vi "Dashboard Main.vi"() -> ()   [LabVIEW 2016]
uses:
  <vilib>/Utility/miscctls.llb/LVRowAndColumnTypeDef.ctl
  <vilib>/event_ctls.llb/eventvkey.ctl
  <vilib>/Utility/file.llb/Read Delimited Spreadsheet (DBL).vi
  <vilib>/Utility/file.llb/Write Delimited Spreadsheet (DBL).vi
  <vilib>/Rock Robotics/Network Tables/NT Write Boolean.vi
  <vilib>/Rock Robotics/Network Tables/NT Read Numeric Array.vi
  <vilib>/Rock Robotics/WPI/Dashboard/WPI_DashboardLogging Global.vi
panel:
  out "error out":errorcluster
  out "error out 2":errorcluster
  in  "Camera Settings Right":T1={"Frame Rate"=30, "Compression"=30, "Size"=1, "DB Camera Config"=FALSE} {"Frame Rate" scale=1.0..30.0; "Compression" scale=100.0..-1.0; "Size" items=["640x480", "320x240", "160x120"]}
  in  "Camera Name Right":string(combo)="No Camera Selection"
  out "Camera Info":cluster{"Mbps LED":bool, "Mbps":dbl, "fps":dbl} {"fps" format="%#.1g"; "Mbps" format="%#.1g"}
  in  "Camera Settings":T1={"Frame Rate"=30, "Compression"=30, "Size"=1, "DB Camera Config"=FALSE} {"Frame Rate" scale=1.0..30.0; "Compression" scale=100.0..-1.0; "Size" items=["640x480", "320x240", "160x120"]}
  in  "TCP":refnum<k5>
  in  "Rec Mode":enum32{"Stop", "Record", "Playback"}(radio)
  out "Robot IP":string
  out "Image Message":string="Timeout in Camera Communications"
  in  "Dashboard Tab":T2(tab)
  in  "Mode":bool
  in  "Select Auto":string(combo)="Select Autonomous ..."
  out "NT Connection":bool
  out "MotorChart R":cluster{"Numeric":dbl, "Numeric":dbl}(graph)
  out "MotorChart L":cluster{"Numeric":dbl, "Numeric":dbl}(graph)
  out "MotorSliders R":cluster{"MotorSlide1":dbl, "MotorSlide2":dbl} {"MotorSlide2" scale=-1.0..1.0 scale format="%#_2e"; "MotorSlide1" scale=-1.0..1.0 scale format="%#_2e"}
  out "MotorSliders L":cluster{"MotorSlide1":dbl, "MotorSlide2":dbl} {"MotorSlide2" scale=-1.0..1.0 scale format="%#_2e"; "MotorSlide1" scale=-1.0..1.0 scale format="%#_2e"}
  out "JS1 Z":dbl(slide) scale=-1.0..1.0 scale format="%#_2e"
  out "JS1 Graph":cluster{"X":dbl, "Y":dbl}[](graph)
  out "JS1 Buttons":T3
  out "JS2 Z":dbl(slide) scale=-1.0..1.0 scale format="%#_2e"
  out "JS2 Graph":cluster{"X":dbl, "Y":dbl}[](graph)
  out "JS2 Buttons":T3
  out "Mode":T4(ring)=enum."Auto Disabled"
  out "Gear State":string="Waiting...."
  out "Camera Image Right":T5(plugin-control)
  in  "Test Slider":dbl(slide) scale=0.0..100.0 scale format="%#_3g"
  in  "On/Off":bool caption="Solenoid"
  in  "Test Name":u16(ring) items=["Select the test to run..."]
  in  "Test Tree":string(tree)
  in  "Motor":cluster{"Value":dbl, "Enable":bool} {"Value" scale=-1.0..1.0 scale format="%#_3g"}
  out "Progress":T6 {"Test Progress" scale=0.0..100.0}
  in  "Rev/Fwd":cluster{"Forward":bool, "Reverse":bool}
  in  "Test Ring":u16(ring) items=["Monochrome", "Color"]
  out "Cmd Status":string
  in  "Execute Command":bool
  in  "Command Params":string[][](table)
  in  "Command Selection":i32(listbox)
  in  "CheckList":i32(listbox)
  out "Tree":string(tree)
  in  "Max Speed":dbl=1.0 format="%#_13g"
  in  "Foreward Sensitivity":dbl=1.0 format="%#_13g"
  in  "Turning Sensitity":dbl=0.4 format="%#_13g"
  in  "High Gear Turning Multiplier":dbl=0.65 format="%#_13g"
  in  "Save":bool
  in  "Load":bool
  in  "Autoshift":bool=TRUE
  in  "Direction Toggle":bool=TRUE
  in  "High Gear":bool=TRUE
  in  "Profile Name":string="Profile1"
  out "Camera Image":T5(plugin-control)
  out "Background":bool
  in  "Camera Name":string(combo)="No Camera Selection"
  # "HW"
  # "HW"
  # "Joysticks"
  # "This is the number that is multiplied with the joystick output to determine high gear turning speed, the lower the number the slower it will turn in high gear."
  # "These numbers controls overall how sensitive the joystick is to turning and foreward movement, the lower the number is the faster it will respond to joystick motion. \nIf the number is 1 then it will move in a linear relationship with the joystick."
  # "This controls the maximum foreward and backwards speed of the robot, if at 1 then the robot can move at max power, if at 0 then the robot cannot move at all."
  # "This turns the ability to use autoshift on/off, if activated it does NOT mean that autoshift is always on, it simply means that it can be turned on with buttons 6/11."
  # "This turns the ability to use high gear on/off, if activated it does NOT mean that high gear is always on, it simply means that it can be turned on with button 1."
  # "This turns on the ability to reverse the direction of the robot with the buttons 8/9."
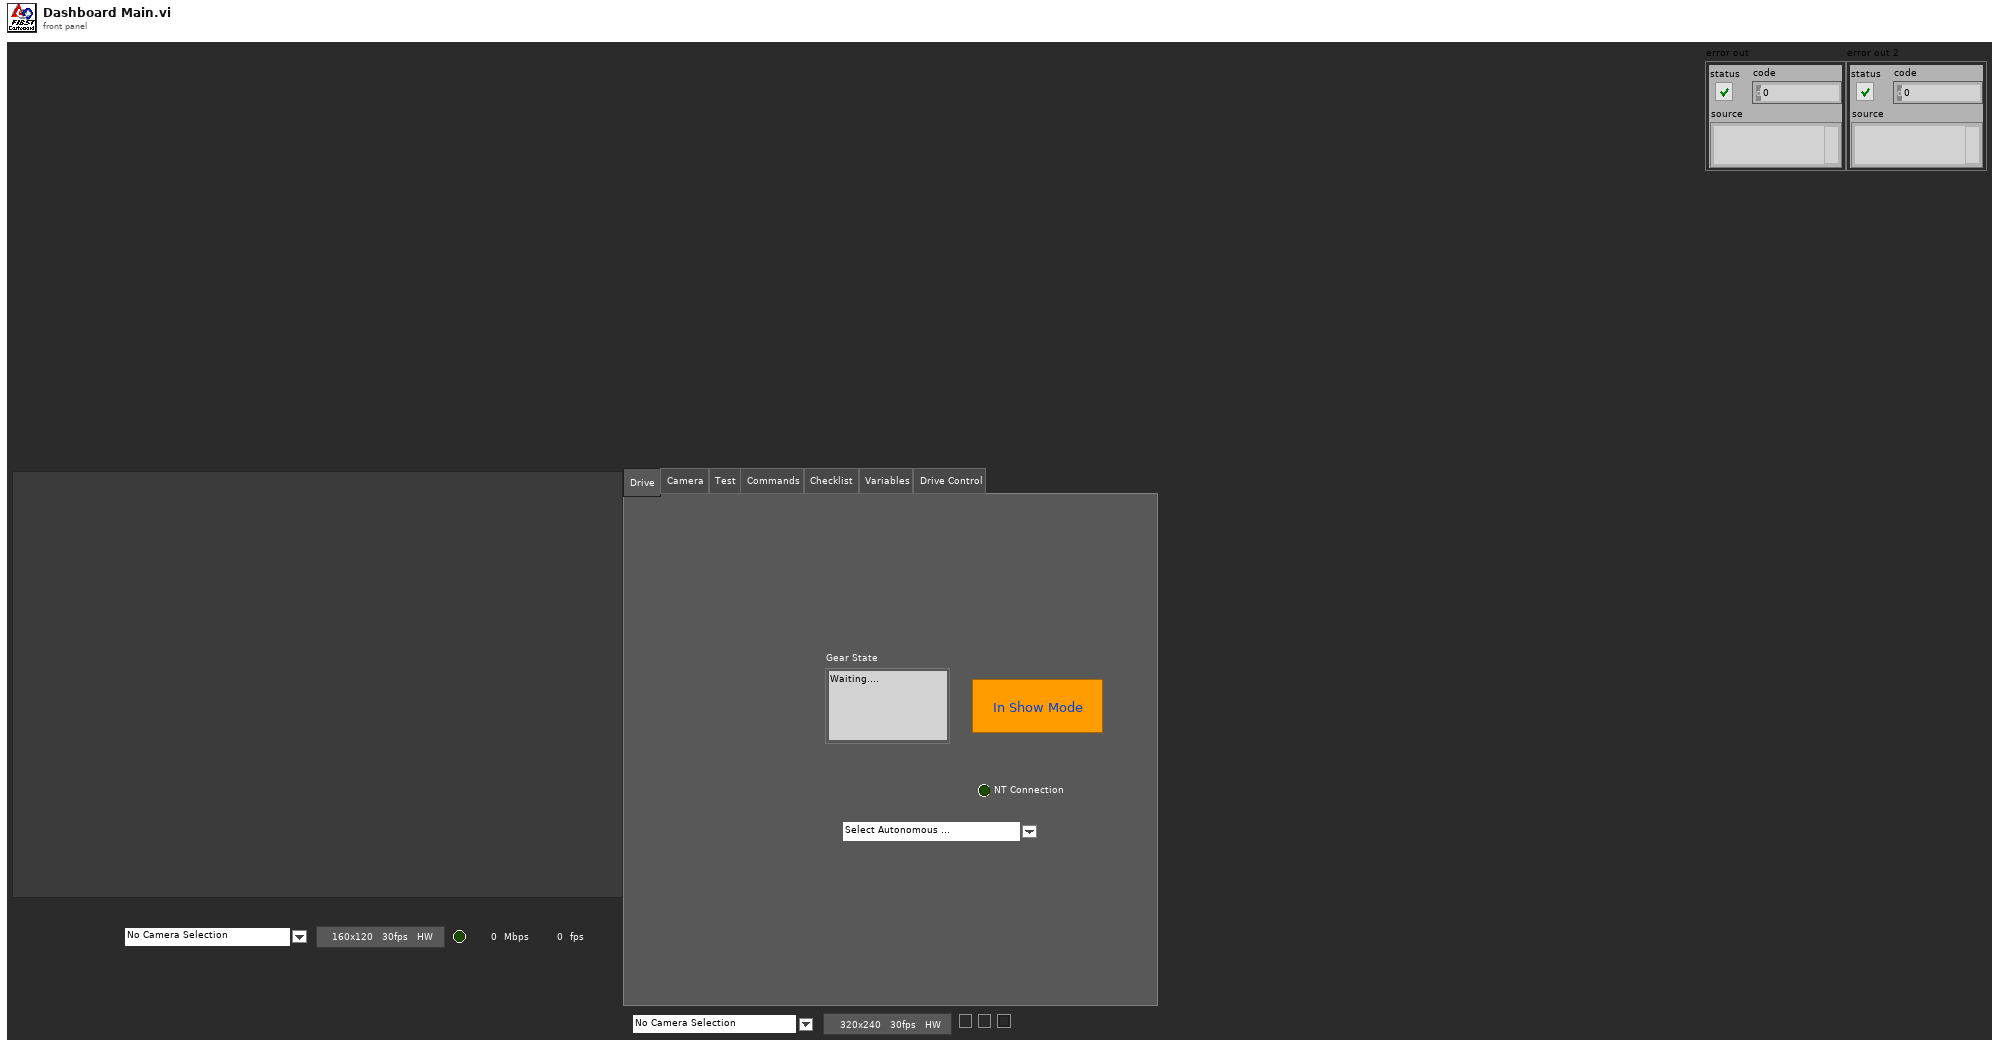
[diagram p1: front panel]
types:
  T1 = cluster{"Frame Rate":i32, "Compression":i32, "Size":u16, "DB Camera Config":bool}
  T2 = enum32{"Drive", "Camera", "Basic", "Custom", "Test", "Commands", "Checklist", "Variables", "Drive Control"}
  T3 = cluster{bool, bool, bool, bool, bool, bool, bool, bool, bool, bool, bool, bool}
  T4 = enum8{"Tele-Op Disabled", "Tele-Op Enabled", "Auto Disabled", "Auto Enabled", "Test Disabled", "Test Enabled", "Disconnected", "No Code", "E-Stop"}
  T5 = typedef "IMAQ Image.ctl" = refnum<image>
  T6 = cluster{"Test Progress":u8, "Test Progress Text":string}
  T7 = typedef "Image Type" = u32
  T8 = cluster{"IDs":cluster{"RPC field ID":u16, "Unique ID":u16}, "String":string}
  T9 = enum32{"Drive", "Camera", "Basic", "Custom", "Test", "Commands", "Checklist", "Variables"}
  T10 = enum32{"Drive", "Basic", "Custom", "Test", "Checklist", "Variables"}
  T11 = cluster{"Error Strings":string, "Disable Counts":cluster{u16, u16}, "Rail Faults":cluster{u16, u16, u16}, "Robot IP":string, "DB Mode":u8, "Event Info":cluster{"Name":string, "Type":u8, "Number":u16, "Replay":u8}}
  T12 = cluster{"Storage":cluster{"Disk Free":u64, "RAM Block":u32, "RAM free":u32}, "CPU Utilization":cluster{"CPU % ISR":sgl, "CPU % Time Crit":sgl, "CPU % Timed Str":sgl, "CPU % High":sgl, "CPU % Above":sgl, "CPU % Normal":sgl, "CPU % Low":sgl}, "CAN":cluster{"% Bus Utilization":sgl, "Bus Off Cnt":u32, "TX_FIFO Full Cnt":u32, "Receive Error Cnt":u8, "Transmit Error Cnt":u8}, "HID":cluster{"HID Outputs":u32, "Rumble Low":u16, "Rumble High":u16}[]}
  T13 = cluster{"Status bits":cluster{"Test Mode":bool, "Autonomous":bool, "Enabled":bool, "Code Start":bool, "Brownout":bool, "Reserved 2":bool, "Reserved 3":bool, "E-Stop":bool}, "Code Trace":cluster{"Disabled":bool, "TeleOp":bool, "Auto":bool, "Test":bool}, "Controller Type":enum16{"unknown", "cRIO", "roboRio"}, "Code?":enum16{"unknown", "noCode", "code"}, "Battery V":dbl}
  T14 = cluster{"Control Bits":cluster{"TestMode":bool, "Autonomous":bool, "Enabled":bool, "FMS Present":bool, bool, bool, bool, "E-Stop":bool}, "Team Station ":u8, "Countdown":sgl, "Joystick Values":cluster{"Axes":dbl[], "Buttons":bool[], "POVs":i16[]}[]}
  T15 = cluster{"Axes":dbl[], "Buttons":bool[], "POVs":i16[]}[]
  T16 = cluster{"Axes":dbl[], "Buttons":bool[], "POVs":i16[]}
  T17 = cluster{"Buttons[0]":bool, "Buttons[1]":bool, "Buttons[2]":bool, "Buttons[3]":bool, "Buttons[4]":bool, "Buttons[5]":bool, "Buttons[6]":bool, "Buttons[7]":bool, "Buttons[8]":bool, "Buttons[9]":bool, "Buttons[10]":bool, "Buttons[11]":bool}
  T18 = cluster{"Camera Image":refnum<vi>, "Dashboard Tab":refnum<vi>, "Background":refnum<vi>, "Rec Mode":refnum<vi>, "Test Slider":refnum<vi>, "On/Off ":refnum<vi>, "Test Ring":refnum<vi>, "Rev/Fwd":refnum<vi>, "Test Name":refnum<vi>, "Motor":refnum<vi>, "Progress":refnum<vi>, "CheckList":refnum<vi>, "Tree":refnum<vi>, "Test Tree":refnum<vi>, "Command Params":refnum<vi>, "Command Selection":refnum<vi>, "Execute Command":refnum<vi>, "Cmd Status":refnum<vi>, "Camera Settings":refnum<vi>, "Camera Name":refnum<vi>, "Camera Info":refnum<vi>, "Camera Settings Right":refnum<vi>, "Camera Name Right":refnum<vi>, "Camera Image Right":refnum<vi>}
  T19 = cluster{"Operation":enum16{"Update", "Clear"}, "Color Box":u32}[]
  T20 = typedef "eventvkey.ctl" = enum16{"ASCII", "Enter", "Return", "Shift", "Ctrl", "Alt", "Cmd", "Opt", "Caps", "NumLock", "Clear", "Break", "Up", "Down", "Left", "Right", "Insert", "Delete", "Home", "End", "PageUp", "PageDown", "Escape", "Help", "Pause", "ScrollLock", "F1", "F2", "F3", "F4", "F5", "F6", "F7", "F8", "F9", "F10", "F11", "F12", "F13", "F14", "F15", "F16", "F17", "F18", "F19", "F20", "F21", "F22", "F23", "F24", "Play", "VolumeUp", "VolumeDown", "Mute", "Two Byte Char"}
  T21 = cluster{"Image Size":bool, "Image Type":bool, "Pixel Value":bool, "ROI Information":bool, "Zoom Factor":bool}
  T22 = cluster{"Operation":enum16{"Update", "Clear"}, "Color Box":u32}
  T23 = typedef "LVRowAndColumnTypeDef.ctl" = cluster{"Row":i32, "Column":i32}
  T24 = cluster{"Shift":bool, "Ctrl":bool, "Alt":bool, "Cmd":bool, "Opt":bool}
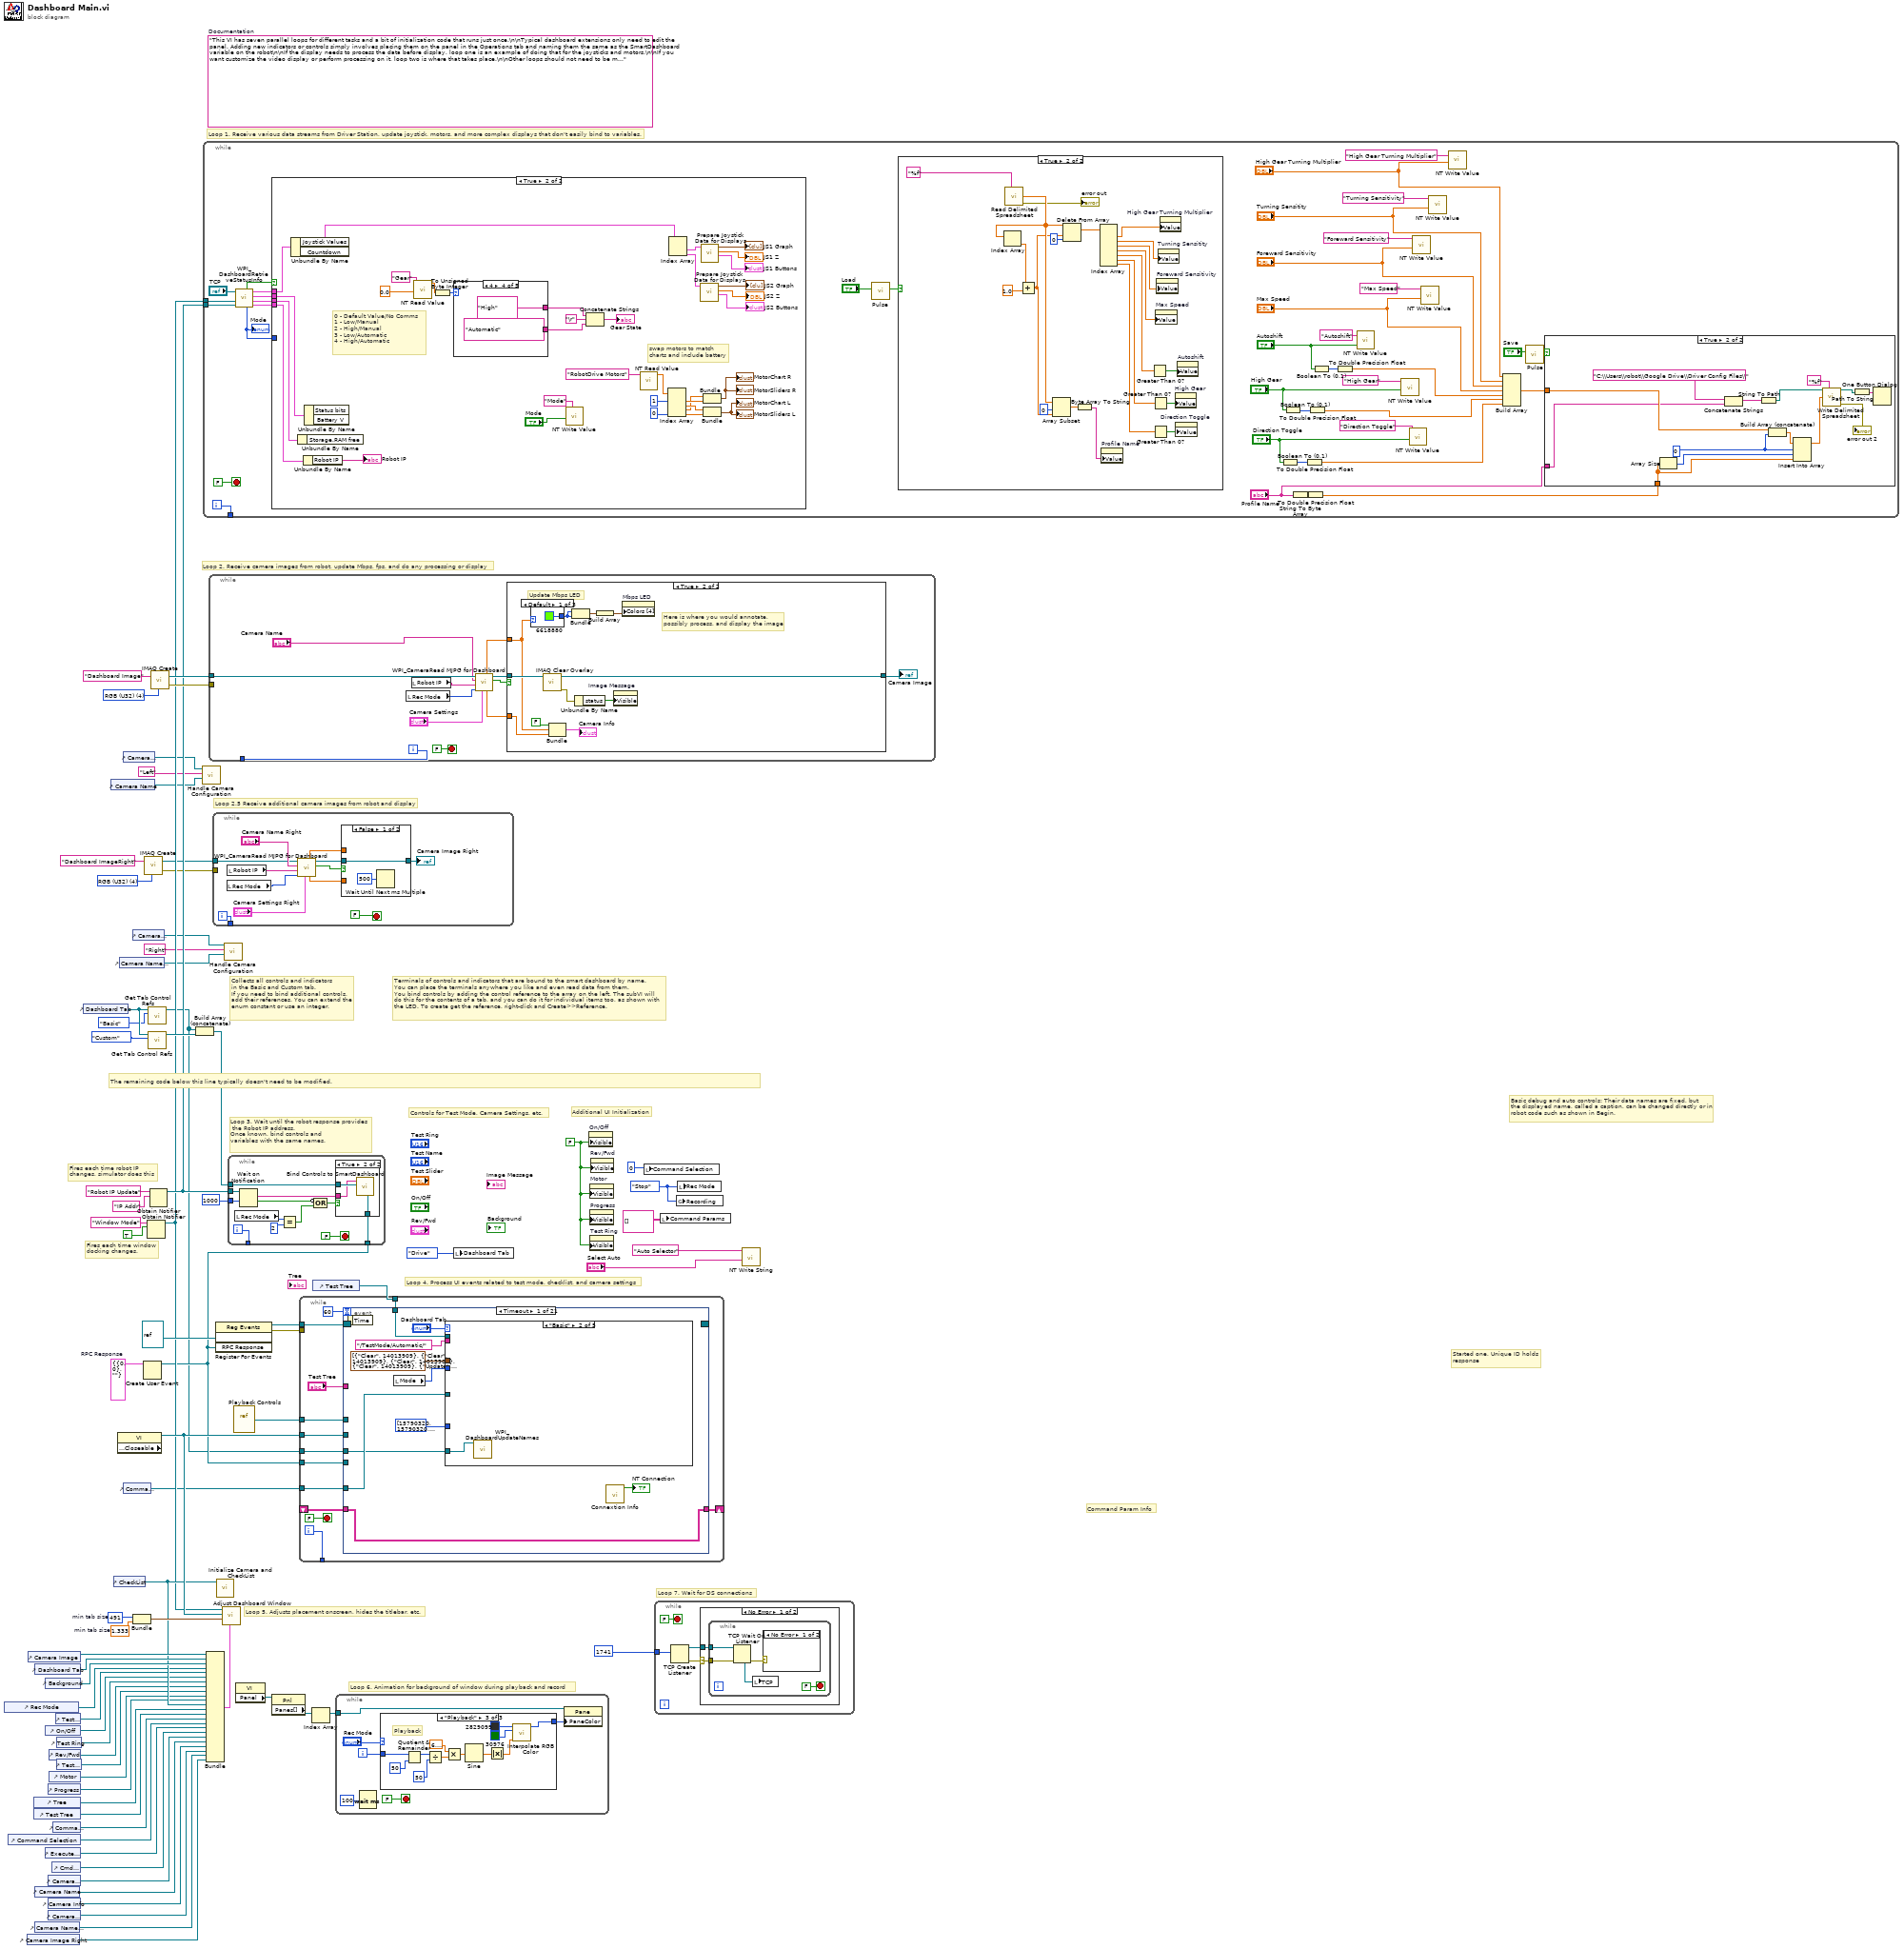
[diagram p0: block diagram]
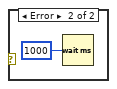
[diagram p3: hidden frame]
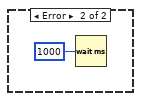
[diagram p4: hidden frame]
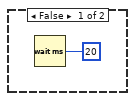
[diagram p7: hidden frame]
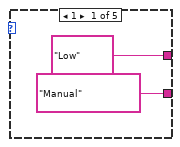
[diagram p8: hidden frame]
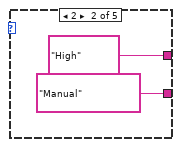
[diagram p9: hidden frame]
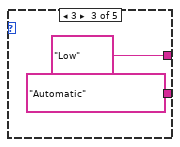
[diagram p10: hidden frame]
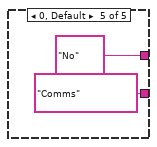
[diagram p11: hidden frame]
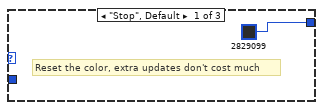
[diagram p12: hidden frame]
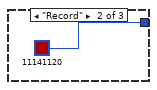
[diagram p13: hidden frame]
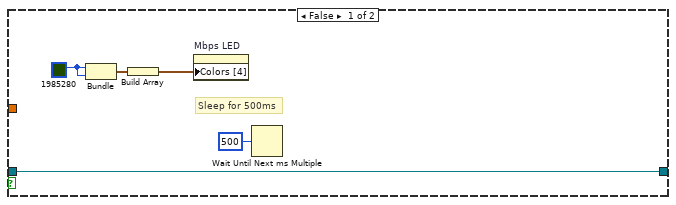
[diagram p15: hidden frame]
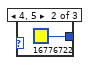
[diagram p16: hidden frame]
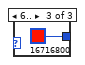
[diagram p17: hidden frame]
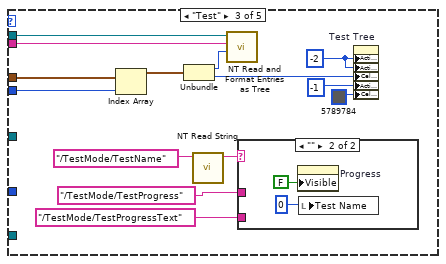
[diagram p19: hidden frame]
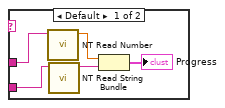
[diagram p20: hidden frame]
diagram:
  w10 = T7 4 items=["Grayscale (U8)", "Grayscale (I16)", "Grayscale (SGL)", "Complex (CSG)", "RGB (U32)", "HSL (U32)", "RGB (U64)"] ("Image Type")
  w26 = T8 {"IDs"={"RPC field ID"=0, "Unique ID"=0}, "String"=""}  # RPC Response
  w51 = 491  # min tab size
  w50 = 1.333  # min tab size
  w58 = enum32{"Stop", "Record", "Playback"}."Stop" ("Rec Mode")
  w33 = FALSE ("Visible")
  (unwired) "This VI has seven parallel loops for different tasks and a bit of initialization code that runs just once.\n\nTypical dashboard extensions only need to edit the panel. Adding new indicators or controls simply involves placing them on the panel in the Operations tab and naming them the same as the SmartDashboard variable on the robot\n\nIf the display needs to process the data before display, loop one is an example of doing that for the joysticks and motors.\n\nIf you want customize the video display or perform processing on it, loop two is where that takes place.\n\nOther loops should not need to be modified. They are pretty standard, and document the task they perform."  # Documentation
  w75 = T7 4 items=["Grayscale (U8)", "Grayscale (I16)", "Grayscale (SGL)", "Complex (CSG)", "RGB (U32)", "HSL (U32)", "RGB (U64)"] ("Image Type")
  # "Loop 2.5 Receive additional camera images from robot and display"
  # "Command Param Info"
  # "Started one, Unique ID holds\nresponse"
  # "Loop 7. Wait for DS connections"
  # "Basic debug and auto controls: Their data names are fixed, but\nthe displayed name, called a caption, can be changed directly or in\nrobot code such as shown in Begin."
  # "Controls for Test Mode, Camera Settings, etc."
  # "Additional UI Initialization"
  # "Loop 6. Animation for background of window during playback and record"
  # "Fires each time robot IP\nchanges, simulator does this"
  # "Fires each time window\ndocking changes."
  # "Collects all controls and indicators\nin the Basic and Custom tab.\nIf you need to bind additional controls,\nadd their references. You can extend the\nenum constant or use an integer."
  # "The remaining code below this line typically doesn't need to be modified."
  # "Loop 4. Process UI events related to test mode, checklist, and camera settings"
  # "Terminals of controls and indicators that are bound to the smart dashboard by name.\nYou can place the terminals anywhere you like and even read data from them.\nYou bind controls by adding the control reference to the array on the left. The subVI will\ndo this for the contents of a tab, and you can do it for individual items too, as shown with\nthe LED. To create get the reference, right-click and Create>>Reference."
  # "Loop 3. Wait until the robot response provides\n the Robot IP address.\nOnce known, bind controls and\nvariables with the same names."
  # "Loop 5. Adjusts placement onscreen, hides the titlebar, etc."
  # "Loop 1. Receive various data streams from Driver Station, update joystick, motors, and more complex displays that don't easily bind to variables."
  # "Loop 2. Receive camera images from robot, update Mbps, fps, and do any processing or display"
  n1 = control-ref of="Rec Mode"() -> (w39:refnum<vi>)
  n2 = control-ref of="Command Selection"() -> (w25:refnum<vi>)
  n3 = control-ref of="Camera Image Right"() -> (w1:refnum<vi>)
  n4 = control-ref of="Camera Image"() -> (w53:refnum<vi>)
  n5 = control-ref of="Tree"() -> (w43:refnum<vi>)
  n6 = control-ref of="Test Tree"() -> (w42:refnum<vi>)
  n7 = control-ref of="Dashboard Tab"() -> (w52:refnum<vi>)
  n8 = control-ref of="Camera Name"() -> (w16:refnum<vi>)
  n9 = control-ref of="Camera Name Right"() -> (w2:refnum<vi>)
  n10 = control-ref of="Execute Command"() -> (w27:refnum<vi>)
  n11 = control-ref of="Background"() -> (w48:refnum<vi>)
  n12 = control-ref of="On/Off"() -> (w37:refnum<vi>)
  n13 = control-ref of="Progress"() -> (w34:refnum<vi>)
  n14 = control-ref of="Camera Settings"() -> (w17:refnum<vi>)
  n15 = control-ref of="Camera Info"() -> (w15:refnum<vi>)
  n16 = control-ref of="Camera Settings Right"() -> (w3:refnum<vi>)
  n17 = control-ref of="Rev/Fwd"() -> (w35:refnum<vi>)
  n18 = control-ref of="Motor"() -> (w40:refnum<vi>)
  n19 = control-ref of="Cmd Status"() -> (w21:refnum<vi>)
  n20 = control-ref of="Command Params"() -> (w28:refnum<vi>)
  n21 = control-ref of="Test Slider"() -> (w38:refnum<vi>)
  n22 = control-ref of="Test Ring"() -> (w36:refnum<vi>)
  n23 = control-ref of="Test Name"() -> (w41:refnum<vi>)
  n24 = control-ref of="Dashboard Tab"() -> (w56:refnum<vi>)
  n25 = control-ref of="Camera Name"() -> (w18:refnum<vi>)
  n26 = control-ref of="CheckList"() -> (w44:refnum<vi>)
  n27 = property class="VI" props=["Front Panel.Closeable"]() -> (reference out=w57:refnum<vi>)  [unwired: 2 in, 2 out]
  n28 = control-ref of="Camera Name Right"() -> (w6:refnum<vi>)
  n29 = control-ref of="Camera Settings"() -> (w19:refnum<vi>)
  n30 = control-ref of="Command Params"() -> (w20:refnum<vi>)
  n31 = control-ref of="Camera Settings Right"() -> (w7:refnum<vi>)
  n32 = Bundle("min tab size"=w51, "min tab size"=w50) -> (w49:cluster{"min tab size":i32, "min tab size":dbl})  [unwired: 1 in]
  n33 = Create User Event(user event datatype=w26) -> (user event=w22:refnum<user-event>)  [unwired: 1 in, 1 out]
  n34 = call "IMAQ Create"("Image Name"="Dashboard ImageRight", "Image Type"=w10) -> ("New Image"=w9:T5, "error out"=w8:errorcluster)  [unwired: 2 in, 1 out]
  n35 = Obtain Notifier(name (unnamed)="Window Mode", notification data type=TRUE) -> (notifier out=w31:refnum<notifier>)  [unwired: 2 in, 2 out]
  n36 = call <vilib>:"Get Tab Control Refs.vi"("Page Index"=T10."Basic" ("Dashboard Tab"), "TabControl in"=w56) -> ("ControlsOnPage"=w14:refnum<vi>[])  [unwired: 9 in]
  n37 = call <vilib>:"Get Tab Control Refs.vi"("Page Index"=T10."Custom" ("Dashboard Tab"), "TabControl in"=w56) -> ("ControlsOnPage"=w55:refnum<vi>[])  [unwired: 9 in]
  n38 = Obtain Notifier(name (unnamed)="Robot IP Update", notification data type="IP Addr" ("name (unnamed)")) -> (notifier out=w32:refnum<notifier>)  [unwired: 2 in, 2 out]
  n39 = call "IMAQ Create"("Image Name"="Dashboard Image", "Image Type"=w75) -> ("New Image"=w73:T5, "error out"=w72:errorcluster)  [unwired: 2 in, 1 out]
  n40 = Build Array (concatenate)(w14, w55) -> (w54:refnum<vi>[])
  n41 = call "Handle Camera Configuration.vi"("CameraNameRef"=w18, "Camera File Name"="Left", "ClusterRef"=w19) -> ()  [unwired: 9 in]
  n42 = while {
    tunnel: [w113] -> _
    tunnel: w32 -> [w107]
    tunnel: w31 -> [w104]
    i -> [w113]
    stop <- FALSE stop-if-true
    n43 = call <vilib>:"WPI_DashboardRetrieveStatusInfo.vi"("Binding Refnum"=w107, "Window Mode Notifier"=w104, "TCP Cnx"="TCP") -> ("Power and Errors"=w108:T11, "Robot Metrics"=w111:T12, "Status Info"=w112:T13, "Control Info"=w109:T14, "Robot Mode"=w106:T4, "Process?"=w110:bool)  [unwired: 3 in]
    "Mode" <- w106
    n44 = case shown="True" w110 {
      tunnel: w112 -> [_ w184]
      tunnel: w111 -> [_ w183]
      tunnel: w109 -> [_ w182]
      tunnel: w108 -> [_ w181]
      tunnel: w106 -> [_ _]
      frame False {
        n45 = Wait (ms)(milliseconds to wait=u32 20) -> ()  [unwired: 1 out]
      }
      frame True {
        # "0 - Default Value/No Comms\n1 - Low/Manual\n2 - High/Manual\n3 - Low/Automatic\n4 - High/Automatic"
        # "swap motors to match\ncharts and include battery"
        n46 = Unbundle By Name(w182) -> ("Joystick Values"=w172:T15)  [unwired: 1 out]
        n47 = Unbundle By Name(w183) -> ()  [unwired: 1 out]
        n48 = Unbundle By Name(w181) -> ("Robot IP"=→"Robot IP":string)
        n49 = Unbundle By Name(w184) -> ()  [unwired: 2 out]
        n50 = call-poly <vilib>:"NT Read Value.vi"("Default Value"=0.0, "Name"="Gear") -> ("Numeric"=w160:dbl)  [unwired: 8 in, 1 out]
        n51 = To Unsigned Byte Integer(number=w160) -> (unsigned 8bit integer=w159:u8)
        n52 = case shown="4" w159 {
          tunnel: ["Low" "High" "Low" "High" "No"] -> w155
          tunnel: ["Manual" "Manual" "Automatic" "Automatic" "Comms"] -> w157
          frame 1 {
          }
          frame 2 {
          }
          frame 3 {
          }
          frame 4 {
          }
          frame 0, Default {
          }
        }
        n53 = call-poly <vilib>:"NT Write Value.vi"("Boolean"="Mode", "Name"="Mode") -> ()  [unwired: 9 in, 1 out]
        n54 = Concatenate Strings(w155, "\r", w157) -> (→"Gear State":string)
        n55 = call-poly <vilib>:"NT Read Value.vi"("Name"="RobotDrive Motors") -> ("Numeric Array"=w162:dbl[])  [unwired: 9 in, 1 out]
        n56 = Index Array(array=w162, index #1=1, index #4=0) -> (element #1=w176:dbl, element #2=w177:dbl, element #3=w175:dbl, element #4=w180:dbl)  [unwired: 2 in]
        n57 = Index Array(array=w172) -> (element #1=w171:T16, element #2=w167:T16)  [unwired: 2 in]
        n58 = call "Prepare Joystick Data for Displays.vi"("Joystick Values"=w167) -> ("Buttons"=→"JS2 Buttons":T17, "Z Axis"=→"JS2 Z":dbl, "Cartesian Data"=→"JS2 Graph":cluster{"X axis":dbl, "X axis":dbl}[])  [unwired: 8 in]
        n59 = call "Prepare Joystick Data for Displays.vi"("Joystick Values"=w171) -> ("Buttons"=→"JS1 Buttons":T17, "Z Axis"=→"JS1 Z":dbl, "Cartesian Data"=→"JS1 Graph":cluster{"X axis":dbl, "X axis":dbl}[])  [unwired: 8 in]
        n60 = Bundle("Numeric"=w175, "Numeric"=w176) -> (→"MotorChart R" →"MotorSliders R":cluster{"Numeric":dbl, "Numeric":dbl})  [unwired: 1 in]
        n61 = Bundle("Numeric"=w177, "Numeric"=w180) -> (→"MotorChart L" →"MotorSliders L":cluster{"Numeric":dbl, "Numeric":dbl})  [unwired: 1 in]
      }
    }
    n62 = call "Pulse.vi"("Input"="Load") -> ("Output"=w94:bool)  [unwired: 10 in]
    n63 = case shown="True" w94 {
      frame False {
      }
      frame True {
        n64 = call-poly <vilib>:"Read Delimited Spreadsheet.vi"("format (%.3f)"="%f") -> ("first row"=w132:dbl[], "error out"=→"error out":errorcluster)  [unwired: 9 in, 4 out]
        n65 = Index Array(array=w132) -> (element=w117:dbl)  [unwired: 1 in]
        n66 = Add(x=w117, y=1.0) -> (x+y=w116:dbl)
        n67 = Array Subset(array=w132, index=0, length=w116) -> (w133:dbl[])
        n68 = Delete From Array(array=w132, length=w116, index=0) -> (array with subset deleted=w130:dbl[])  [unwired: 1 out]
        n69 = Byte Array To String(unsigned byte array=w133) -> (string=w119:string)
        n70 = Index Array(array=w130) -> (element #1=w129:dbl, element #2=w128:dbl, element #3=w127:dbl, element #4=w126:dbl, element #5=w125:dbl, element #6=w124:dbl, element #7=w123:dbl)  [unwired: 7 in]
        n71 = property on="Profile Name" class="Str"("Value"=w119) -> ()  [unwired: 2 in, 2 out]
        n72 = Greater Than 0?(x=w125) -> (x > 0?=w120:bool)
        n73 = Greater Than 0?(x=w124) -> (x > 0?=w121:bool)
        n74 = Greater Than 0?(x=w123) -> (x > 0?=w122:bool)
        n75 = property on="Max Speed" class="DigNum (strict)"("Value"=w126) -> ()  [unwired: 2 in, 2 out]
        n76 = property on="Foreward Sensitivity" class="DigNum (strict)"("Value"=w127) -> ()  [unwired: 2 in, 2 out]
        n77 = property on="Turning Sensitity" class="DigNum (strict)"("Value"=w128) -> ()  [unwired: 2 in, 2 out]
        n78 = property on="High Gear Turning Multiplier" class="DigNum (strict)"("Value"=w129) -> ()  [unwired: 2 in, 2 out]
        n79 = property on="High Gear" class="Bool (strict)"("Value"=w121) -> ()  [unwired: 2 in, 2 out]
        n80 = property on="Direction Toggle" class="Bool (strict)"("Value"=w122) -> ()  [unwired: 2 in, 2 out]
        n81 = property on="Autoshift" class="Bool (strict)"("Value"=w120) -> ()  [unwired: 2 in, 2 out]
      }
    }
    n82 = Boolean To (0,1)(Boolean="Direction Toggle") -> (0, 1=w97:i16)
    n83 = Boolean To (0,1)(Boolean="High Gear") -> (0, 1=w99:i16)
    n84 = String To Byte Array(string="Profile Name") -> (unsigned byte array=w93:u8[])
    n85 = To Double Precision Float(number=w97) -> (double precision float=w96:dbl)
    n86 = To Double Precision Float(number=w93) -> (double precision float=w91:dbl[])
    n87 = To Double Precision Float(number=w99) -> (double precision float=w98:dbl)
    n88 = Boolean To (0,1)(Boolean="Autoshift") -> (0, 1=w101:i16)
    n89 = To Double Precision Float(number=w101) -> (double precision float=w100:dbl)
    n90 = call-poly <vilib>:"NT Write Value.vi"("Boolean"="Autoshift", "Name"="Autoshift") -> ()  [unwired: 9 in, 1 out]
    n91 = call-poly <vilib>:"NT Write Value.vi"("Boolean"="High Gear", "Name"="High Gear") -> ()  [unwired: 9 in, 1 out]
    n92 = call-poly <vilib>:"NT Write Value.vi"("Boolean"="Direction Toggle", "Name"="Direction Toggle") -> ()  [unwired: 9 in, 1 out]
    n93 = call-poly <vilib>:"NT Write Value.vi"("Numeric"="Foreward Sensitivity", "Name"="Foreward Sensitivity") -> ()  [unwired: 9 in, 1 out]
    n94 = call-poly <vilib>:"NT Write Value.vi"("Numeric"="Max Speed", "Name"="Max Speed") -> ()  [unwired: 9 in, 1 out]
    n95 = call-poly <vilib>:"NT Write Value.vi"("Numeric"="Turning Sensitity", "Name"="Turning Sensitivity") -> ()  [unwired: 9 in, 1 out]
    n96 = call-poly <vilib>:"NT Write Value.vi"("Numeric"="High Gear Turning Multiplier", "Name"="High Gear Turning Multiplier") -> ()  [unwired: 9 in, 1 out]
    n97 = Build Array("High Gear Turning Multiplier", "Turning Sensitity", "Foreward Sensitivity", "Max Speed", w100, w98, w96) -> (w92:dbl[])
    n98 = call "Pulse.vi"("Input"="Save") -> ("Output"=w102:bool)  [unwired: 10 in]
    n99 = case shown="True" w102 {
      tunnel: w92 -> [_ w145]
      tunnel: w91 -> [_ w147]
      tunnel: "Profile Name" -> [_ w141]
      frame False {
      }
      frame True {
        w144 = 0 ("index")
        n100 = Array Size(array=w147) -> (size(s)=w148:i32)
        n101 = Concatenate Strings("C:\\Users\\robot\\Google Drive\\Driver Config Files\\" ("string"), w141) -> (w140:string)
        n102 = String To Path(string=w140) -> (path=w139:path)
        n103 = Build Array (concatenate)(w145, w144) -> (w143:dbl[])
        n104 = Insert Into Array(array=w143, index=w144, new element #1=w148, new element #2=w147) -> (w146:dbl[])
        n105 = call-poly <vilib>:"Write Delimited Spreadsheet.vi"("file path (dialog if empty)"=w139, "format (%.3f)"="%f", "1D data"=w146) -> ("new file path (Not A Path if cancelled)"=w137:path, "error out"=→"error out 2":errorcluster)  [unwired: 11 in]
        n106 = Path To String(path=w137) -> (string=w138:string)
        n107 = One Button Dialog(message=w138) -> ()  [unwired: 1 in, 1 out]
      }
    }
  }
  n108 = Bundle("Camera Image"=w53, "Dashboard Tab"=w52, "Background"=w48, "Rec Mode"=w39, "Test Slider"=w38, "On/Off"=w37, "Test Ring"=w36, "Rev/Fwd"=w35, "Test Name"=w41, "Motor"=w40, "Progress"=w34, "CheckList"=w44, "Tree"=w43, "Test Tree"=w42, "Command Params"=w28, "Command Selection"=w25, "Execute Command"=w27, "Cmd Status"=w21, "Camera Settings"=w17, "Camera Name"=w16, "Camera Info"=w15, "Camera Settings Right"=w3, "Camera Name Right"=w2, "Camera Image Right"=w1) -> (w45:T18)  [unwired: 1 in]
  n109 = while {
    tunnel: w73 -> [w204]
    tunnel: w72 -> [_]
    tunnel: [w205] -> _
    i -> [w205]
    stop <- FALSE stop-if-true
    n110 = local read "Rec Mode"() -> (w200:enum32{"Stop", "Record", "Playback"})
    n111 = local read "Robot IP"() -> (w199:string)
    n112 = call <vilib>:"WPI_CameraRead MJPG for Dashboard.vi"("Camera Settings"="Camera Settings", "Rec Mode"=w200, "Robot IP"=w199, "Camera Name"="Camera Name", "Refnum in"=w204) -> ("Active"=w202:bool, "Refnum out"=w203:T5, "FPS"=w201:dbl, "Bandwidth (Mbps)"=w198:dbl)  [unwired: 3 in]
    n113 = case shown="True" w202 {
      tunnel: w203 -> [w207 w218]
      tunnel: w198 -> [_ w215]
      tunnel: w201 -> [_ w216]
      tunnel: [w207 w212] -> w196
      frame False {
        w209 = u32 1985280 ("Color Box")
        # "Sleep for 500ms"
        n114 = Bundle("Color Box"=w209, "Color Box"=w209) -> (w210:cluster{"Color Box":u32, "Color Box":u32})  [unwired: 1 out]
        n115 = Build Array(w210) -> (w208:cluster{"Color Box":u32, "Color Box":u32}[])
        n116 = property on="Mbps LED" class="Bool (strict)"("Colors [4]"=w208) -> ()  [unwired: 2 in, 2 out]
        n117 = Wait Until Next ms Multiple(millisecond multiple=u32 500) -> ()  [unwired: 1 out]
      }
      frame True {
        # "Here is where you would annotate,\npossibly process, and display the image"
        # "Update Mbps LED"
        n118 = case shown="Default" w215 {
          tunnel: [u32 6618880 ("Color Box") u32 16776722 ("Color Box") u32 16716800 ("Color Box")] -> w219
          frame Default {
          }
          frame 4, 5 {
          }
          frame 6.. {
          }
        }
        n119 = call "IMAQ Clear Overlay"("Image"=w218) -> ("error out"=w221:errorcluster, "Image Out"=w212:T5)  [unwired: 2 in, 7 out]
        n120 = Bundle(FALSE, "Bandwidth (Mbps)"=w215, "FPS"=w216) -> (→"Camera Info":cluster{bool, "Bandwidth (Mbps)":dbl, "FPS":dbl})  [unwired: 1 in]
        n121 = Bundle("Color Box"=w219, "Color Box"=w219) -> (w220:cluster{"Color Box":u32, "Color Box":u32})  [unwired: 1 out]
        n122 = Unbundle By Name(w221) -> ("status"=w222:bool)
        n123 = Build Array(w220) -> (w217:cluster{"Color Box":u32, "Color Box":u32}[])
        n124 = property on="Image Message" class="Str"("Visible"=w222) -> ()  [unwired: 2 in, 2 out]
        n125 = property on="Mbps LED" class="Bool (strict)"("Colors [4]"=w217) -> ()  [unwired: 2 in, 2 out]
      }
    }
    "Camera Image" <- w196
  }
  n126 = while {
    tunnel: w9 -> [w236]
    tunnel: w8 -> [_]
    tunnel: [w230] -> _
    i -> [w230]
    stop <- FALSE stop-if-true
    n127 = local read "Rec Mode"() -> (w234:enum32{"Stop", "Record", "Playback"})
    n128 = local read "Robot IP"() -> (w235:string)
    n129 = call <vilib>:"WPI_CameraRead MJPG for Dashboard.vi"("Camera Settings"="Camera Settings Right", "Rec Mode"=w234, "Robot IP"=w235, "Camera Name"="Camera Name Right", "Refnum in"=w236) -> ("Active"=w229:bool, "Refnum out"=w232:T5, "FPS"=w227:dbl, "Bandwidth (Mbps)"=w228:dbl)  [unwired: 3 in]
    n130 = case shown="False" w229 {
      tunnel: w232 -> [w238 w240]
      tunnel: w228 -> [_ _]
      tunnel: w227 -> [_ _]
      tunnel: [w238 w240] -> w226
      frame False {
        n131 = Wait Until Next ms Multiple(millisecond multiple=u32 500) -> ()  [unwired: 1 out]
      }
      frame True {
      }
    }
    "Camera Image Right" <- w226
  }
  n132 = register-events(refnum<vi> refnum, w22) -> (reference out=w62:refnum<event-registration>, error out=w61:errorcluster)  [unwired: 2 in]
  n133 = call "Initialize Camera and CheckList.vi"("ListBox in"=w44) -> ()  [unwired: 11 in]
  n134 = call "Adjust Dashboard Window.vi"("Sizing Refnums"=w45, "Size Constraints"=w49, "VI"=w57, "WIn Mode"=w31) -> ()  [unwired: 8 in]
  n135 = call "Handle Camera Configuration.vi"("CameraNameRef"=w6, "Camera File Name"="Right", "ClusterRef"=w7) -> ()  [unwired: 9 in]
  n136 = while {
    tunnel: w54 -> [w252]
    tunnel: w32 -> [w250]
    tunnel: [w248] -> _
    tunnel: u32 1000 ("milliseconds to wait") -> [w247]
    tunnel: w22 -> [w241]
    i -> [w248]
    stop <- FALSE stop-if-true
    n137 = local read "Rec Mode"() -> (w243:enum32{"Stop", "Record", "Playback"})
    n138 = Wait on Notification(notifier=w250, timeout in ms (-1)=w247) -> (notification=w249:string, timed out?=w245:bool)  [unwired: 2 in, 2 out]
    n139 = Equal?(x=w243, y=u16 2 ("Rec Mode")) -> (x = y?=w244:bool)
    n140 = Compound Arithmetic op=OR(invert w245, w244) -> (w246:bool)
    n141 = case shown="True" w246 {
      tunnel: w252 -> [_ w255]
      tunnel: w249 -> [_ w254]
      tunnel: w241 -> [_ w253]
      frame False {
      }
      frame True {
        n142 = call <vilib>:"Bind Controls to SmartDashboard.vi"("RPC ref"=w253, "Bound Control Refs"=w255, "Server IP Address"=w254) -> ()  [unwired: 9 in]
      }
    }
  }
  n143 = vi-ref "Playback Controls.vi"() -> (w63:refnum<vi>)
  n144 = property class="VI"() -> ("Panel"=w65:refnum<vi>)  [unwired: 2 in, 2 out]
  n145 = property class="Pnl"(reference=w65) -> ("Panes[]"=w66:refnum<vi>[])  [unwired: 1 in, 2 out]
  n146 = Index Array(array=w66) -> (element=w64:refnum<vi>)  [unwired: 1 in]
  n147 = control-ref of="Test Tree"() -> (w67:refnum<vi>)
  n148 = while {
    tunnel: [w265] -> _
    tunnel: w67 -> [w264]
    tunnel: w63 -> [w263]
    tunnel: w62 -> [w262]
    tunnel: w61 -> [_]
    tunnel: w57 -> [w261]
    tunnel: w22 -> [w260]
    tunnel: w20 -> [w259]
    shift-right: [w258] -> _
    shift-left: _ -> [w257]
    tunnel: w14 -> [w256]
    i -> [w265]
    stop <- FALSE stop-if-true
    n149 = event shown="[0] Timeout" {
      selector: w262 -> [_ _ _ _ _ _ _ _ _ _ _ _ _ _ _ _ _ _ _ _ _]
      dyn-events: [_ _ _ _ _ _ _ _ _ _ _ _ _ _ _ _ w526 _ _ _ _] -> _
      timeout: u32 60 ("milliseconds to wait") -> [_ _ _ _ _ _ _ _ _ _ _ _ _ _ _ _ _ _ _ _ _]
      tunnel: w264 -> [w277 _ _ _ _ _ _ _ _ _ _ _ _ _ _ _ _ _ _ _ _]
      tunnel: "Test Tree" -> [_ _ _ _ _ _ _ _ _ _ _ w488 w500 w503 w507 w515 _ _ _ _ _]
      tunnel: w263 -> [_ _ _ _ _ _ _ _ _ _ _ _ _ _ _ _ w528 _ w546 _ _]
      tunnel: w261 -> [_ _ _ _ _ _ _ _ _ _ _ _ _ _ _ _ w524 _ _ _ _]
      tunnel: w260 -> [_ _ _ _ _ _ _ _ _ _ _ _ _ _ _ _ w520 _ _ _ _]
      tunnel: w259 -> [w272 _ _ _ _ _ w439 _ _ _ _ _ _ _ _ _ _ _ _ _ _]
      tunnel: [w271 w316 w418 w423 w432 w436 w437 w446 w456 w463 w475 w487 w501 w502 w506 w514 w519 w541 w543 w547 w558] -> w258
      tunnel: w257 -> [w271 w316 w418 w423 w432 w436 w437 _ _ w463 w475 w487 w501 w502 w506 w514 w519 w541 w543 w547 w558]
      tunnel: w256 -> [w269 _ _ _ _ _ _ _ _ _ _ _ _ _ _ _ _ _ _ _ _]
      event Timeout {
        n150 = event-data() -> ()  [unwired: 1 in, 1 out]
        n151 = local read "Mode"() -> (w274:T4)
        n152 = case shown="\"Basic\"" "Dashboard Tab" {
          tunnel: w277 -> [_ _ w293 _ _]
          tunnel: "/TestMode/Automatic/" ("Name Pattern") -> [_ _ w292 _ _]
          tunnel: T19 [{"Operation"=enum."Clear", "Color Box"=14013909}, {"Operation"=enum."Clear", "Color Box"=14013909}, {"Operation"=enum."Clear", "Color Box"=14013909}, {"Operation"=enum."Clear", "Color Box"=14013909}, {"Operation"=enum."Update", "Color Box"=14013909}, {"Operation"=enum."Update", "Color Box"=16777215}, {"Operation"=enum."Clear", "Color Box"=14013909}, {"Operation"=enum."Clear", "Color Box"=14013909}, {"Operation"=enum."Clear", "Color Box"=14013909}] -> [_ _ w285 _ w309]
          tunnel: w274 -> [_ _ w284 _ w308]
          tunnel: u32[] [15790320, 15790320, 15790320, 15790320, 16777215, 16777215, 15790320, 15790320, 15790320] -> [_ _ _ _ w314]
          tunnel: w272 -> [_ _ _ _ w302]
          tunnel: w269 -> [_ w279 _ _ _]
          frame "Custom", Default {
          }
          frame "Basic" {
            n153 = call <vilib>:"WPI_DashboardUpdateNames.vi"("Controls on Tab"=w279) -> ()  [unwired: 11 in]
          }
          frame "Test" {
            w291 = -2 ("Active Item:Row Number")
            n154 = Index Array(array=w285, index=w284) -> (element=w286:T22)
            n155 = Unbundle(w286) -> ("Operation"=w287:enum16{"Update", "Clear"}, "Color Box"=w288:u32)
            n156 = call <vilib>:"NT Read String.vi"("Name"="/TestMode/TestName") -> ("String"=w282:string)  [unwired: 9 in, 1 out]
            n157 = call <vilib>:"NT Read and Format Entries as Tree.vi"("Operation"=w287, "Name Pattern"=w292, "Tree Refnum"=w293) -> ()  [unwired: 7 in, 2 out]
            n158 = case shown="\"\"" w282 {
              tunnel: "/TestMode/TestProgress" ("Name") -> [w295 _]
              tunnel: "/TestMode/TestProgressText" ("Name") -> [w294 _]
              frame Default {
                n159 = call <vilib>:"NT Read Number.vi"("Name"=w295) -> ("Numeric"=w296:dbl)  [unwired: 9 in, 1 out]
                n160 = call <vilib>:"NT Read String.vi"("Name"=w294) -> ("String"=w297:string)  [unwired: 9 in, 1 out]
                n161 = Bundle("Numeric"=w296, "String"=w297) -> (→"Progress":cluster{"Numeric":dbl, "String":string})  [unwired: 1 in]
              }
              frame "" {
                n162 = property on="Progress" class="Clust (strict)"("Visible"=FALSE) -> ()  [unwired: 2 in, 2 out]
                n163 = local write "Test Name"(u16 0) -> ()
              }
            }
            n164 = property on="Test Tree" class="Tree (strict)"("Active Item Row Number"=w291, "ActiveColNum"=w291, "CellBG"=w288, "Active Item Row Number"=-1 ("Active Item:Row Number"), "CellBG"=u32 5789784 ("Color Box")) -> ()  [unwired: 2 in, 2 out]
          }
          frame "Variables" {
            n165 = control-ref of="Tree"() -> (w301:refnum<vi>)
            n166 = call <vilib>:"NT Read and Format Entries as Tree.vi"("Tree Refnum"=w301) -> ()  [unwired: 9 in, 2 out]
          }
          frame "Commands" {
            w310 = u32 5789784 ("Color Box")
            w311 = T23 {"Row"=-1, "Column"=-2} ("Active Cell:Active Cell")
            w313 = T23 {"Row"=-2, "Column"=-2} ("Active Cell:Active Cell")
            n167 = Index Array(array=w314, index=w308) -> (element=w312:u32)
            n168 = Index Array(array=w309, index=w308) -> (element=w307:T22)
            n169 = Unbundle(w307) -> ("Operation"=w306:enum16{"Update", "Clear"})  [unwired: 1 out]
            n170 = local read "Command Selection"() -> (w305:i32)
            n171 = property on="Command Selection" class="MCListbox (strict)"("ActiveCell"=w313, "CellBG"=w312, "ActiveCell"=w311, "CellBG"=w310) -> ()  [unwired: 2 in, 2 out]
            n172 = call <vilib>:"WPI_DashboardUpdate RPC Info.vi"("Operation"=w306) -> ("update"=w304:bool, "commands"=w303:string[][])  [unwired: 9 in]
            n173 = property on="Command Selection" class="MCListbox (strict)"("ItemNames"=w303) -> ()  [unwired: 2 in, 2 out]
            n174 = property on="Command Params" class="Tbl (strict)"("Active Cell"=w313, "Cell BG Color"=w312, "Active Cell"=w311, "Cell BG Color"=w310) -> ()  [unwired: 2 in, 2 out]
            n175 = call <vilib>:"WPI_DashboardUpdate Command Params.vi"("Update"=w304, "NewVal"=w305, "Commands"=w303, "Param Tbl"=w302) -> ()  [unwired: 7 in, 1 out]
          }
        }
        n176 = call <vilib>:"Connextion Info.vi"() -> ("Connected"=→"NT Connection":bool)  [unwired: 10 in, 1 out]
      }
      event "Test Tree": Value Change {
        # "Show appropriate\ncontrols"
        n177 = event-data() -> ("CtlRef"=w319:refnum<vi>, "NewVal"=w317:string)  [unwired: 1 in]
        n178 = call <vilib>:"WPI_UtilitiesGetTreeIOName.vi"("NewVal"=w317, "TreeControl in"=w319) -> ("I/O Name"=w320:string)  [unwired: 9 in]
        n179 = case shown="\"Camera\"" w320 {
          selector: w320 -> [_ w327 _ w349 w358 _]
          tunnel: w317 -> [_ _ w346 w348 _ w365]
          tunnel: cluster{string[]}[] [{["640x480", "320x240", "160x120"]}, {["Auto", "Fixed indoor", "Fixed outdoor 1", "Fixed outdoor 2", "Fixed fluorescent 1", "Fixed fluorescent 2", "Hold current"]}, {["Auto", "Flicker-free 50 Hz", "Flicker-free 60 Hz", "Hold current"]}, {["None", "Prioritize frame rate", "Prioritize image quality"]}, {["Monochrome", "Color"]}] -> [_ _ _ _ _ w364]
          frame Default {
            w322 = FALSE ("Visible")
            w321 = FALSE ("Visible")
            n180 = property on="Motor" class="Clust (strict)"("Visible"=w321) -> ()  [unwired: 2 in, 2 out]
            n181 = property on="Test Ring" class="Ring (strict)"("Visible"=w321) -> ()  [unwired: 2 in, 2 out]
            n182 = property on="Rev/Fwd" class="Clust (strict)"("Visible"=w322) -> ()  [unwired: 2 in, 2 out]
            n183 = property on="On/Off" class="Bool (strict)"("Visible"=w322) -> ()  [unwired: 2 in, 2 out]
            n184 = property on="Test Slider" class="Slide (strict)"("Visible"=w322) -> ()  [unwired: 2 in, 2 out]
          }
          frame "Analog Out", "Motor", "PWM" {
            w328 = FALSE ("Visible")
            n185 = case shown="\"Analog Out\"" w327 {
              tunnel: [1.0 ("Value") -1.0 ("Value") 0.0 ("Value")] -> w326
              tunnel: [255.0 ("Value") 1.0 ("Value") 5.0 ("Value")] -> w325
              tunnel: [128.0 ("Value") 0.0 ("Value") 0.0 ("Value")] -> w324
              tunnel: [64.0 ("Value") 0.5 ("Value") 1.0 ("Value")] -> w323
              frame "PWM" {
              }
              frame "Motor", Default {
              }
              frame "Analog Out" {
              }
            }
            n186 = property on="Motor" class="Clust (strict)"("Visible"=TRUE) -> ()  [unwired: 2 in, 2 out]
            n187 = property on="Value" class="Slide (strict)"("Value"=w324, "Scale.Minimum"=w326, "Scale.Maximum"=w325, "Scale.Increment"=w323) -> ()  [unwired: 2 in, 2 out]
            n188 = property on="On/Off" class="Bool (strict)"("Visible"=w328) -> ()  [unwired: 2 in, 2 out]
            n189 = property on="Test Slider" class="Slide (strict)"("Visible"=w328) -> ()  [unwired: 2 in, 2 out]
            n190 = property on="Test Ring" class="Ring (strict)"("Visible"=w328) -> ()  [unwired: 2 in, 2 out]
            n191 = property on="Rev/Fwd" class="Clust (strict)"("Visible"=w328) -> ()  [unwired: 2 in, 2 out]
          }
          frame "Servo" {
            w344 = FALSE ("Visible")
            n192 = call <vilib>:"NT Read Number.vi"("Name"=w346) -> ("Numeric"=w345:dbl)  [unwired: 9 in, 1 out]
            n193 = property on="Test Slider" class="Slide (strict)"("Visible"=TRUE, "Scale.Maximum"=170.0 ("Scale.Range:Maximum")) -> ()  [unwired: 2 in, 2 out]
            n194 = local write "Test Slider"(w345) -> ()
            n195 = property on="Motor" class="Clust (strict)"("Visible"=w344) -> ()  [unwired: 2 in, 2 out]
            n196 = property on="Rev/Fwd" class="Clust (strict)"("Visible"=w344) -> ()  [unwired: 2 in, 2 out]
            n197 = property on="On/Off" class="Bool (strict)"("Visible"=w344) -> ()  [unwired: 2 in, 2 out]
            n198 = property on="Test Ring" class="Ring (strict)"("Visible"=w344) -> ()  [unwired: 2 in, 2 out]
          }
          frame "Relay", "Solenoid" {
            w347 = FALSE ("Visible")
            n199 = property on="Motor" class="Clust (strict)"("Visible"=w347) -> ()  [unwired: 2 in, 2 out]
            n200 = property on="Test Slider" class="Slide (strict)"("Visible"=w347) -> ()  [unwired: 2 in, 2 out]
            n201 = Search and Replace String(input string=w348, search string="/Value  **", replace string="/Direction") -> (result string=w354:string)  [unwired: 5 in, 3 out]
            n202 = property on="Test Ring" class="Ring (strict)"("Visible"=w347) -> ()  [unwired: 2 in, 2 out]
            n203 = call <vilib>:"NT Read String.vi"("Name"=w354) -> ("String"=w352:string)  [unwired: 9 in, 1 out]
            n204 = Equal?(x="Both directions", y=w352) -> (x = y?=w350:bool)
            n205 = Not(x=w350) -> (.not. x?=w351:bool)
            n206 = property on="Rev/Fwd" class="Clust (strict)"("Visible"=w350) -> ()  [unwired: 2 in, 2 out]
            n207 = property on="On/Off" class="Bool (strict)"("Visible"=w351, "Caption.Text"=w349) -> ()  [unwired: 2 in, 2 out]
          }
          frame "Compressor", "Digital Out" {
            w357 = FALSE ("Visible")
            # "Get direction and finish"
            n208 = property on="Motor" class="Clust (strict)"("Visible"=w357) -> ()  [unwired: 2 in, 2 out]
            n209 = property on="Test Slider" class="Slide (strict)"("Visible"=w357) -> ()  [unwired: 2 in, 2 out]
            n210 = property on="Test Ring" class="Ring (strict)"("Visible"=w357) -> ()  [unwired: 2 in, 2 out]
            n211 = property on="On/Off" class="Bool (strict)"("Visible"=TRUE, "Caption.Text"=w358) -> ()  [unwired: 2 in, 2 out]
            n212 = property on="Rev/Fwd" class="Clust (strict)"("Visible"=FALSE) -> ()  [unwired: 2 in, 2 out]
          }
          frame "Camera" {
            n213 = call <vilib>:"Get Last Path Segment.vi"("String in"=w365) -> ("String out"=w366:string)  [unwired: 10 in]
            n214 = property on="On/Off" class="Bool (strict)"("Visible"=FALSE) -> ()  [unwired: 2 in, 2 out]
            n215 = property on="Motor" class="Clust (strict)"("Visible"=FALSE) -> ()  [unwired: 2 in, 2 out]
            n216 = property on="Rev/Fwd" class="Clust (strict)"("Visible"=FALSE) -> ()  [unwired: 2 in, 2 out]
            n217 = case shown="\"White Balance  **\"" w366 {
              tunnel: w365 -> [w372 w381 w390 w399 w408 _ w414]
              tunnel: w364 -> [w370 w378 w387 w396 w405 _ _]
              frame "Size  **" {
                n218 = Index Array(array=w370) -> (element=w369:cluster{string[]})  [unwired: 1 in]
                n219 = call <vilib>:"NT Read String.vi"("Name"=w372) -> ("String"=w371:string)  [unwired: 9 in, 1 out]
                n220 = Unbundle(w369) -> (w367:string[])
                n221 = Match First String(2:w367, 3:w371) -> (0:w368:i32)  [unwired: 1 out]
                n222 = property on="Test Ring" class="Ring (strict)"("Value"=w368, "Strings []"=w367) -> ()  [unwired: 2 in, 2 out]
                n223 = property on="Test Ring" class="Ring (strict)"("Visible"=TRUE) -> ()  [unwired: 2 in, 2 out]
                n224 = property on="Test Slider" class="Slide (strict)"("Visible"=FALSE) -> ()  [unwired: 2 in, 2 out]
              }
              frame "White Balance  **" {
                n225 = Index Array(array=w378, index=1) -> (element=w379:cluster{string[]})
                n226 = call <vilib>:"NT Read String.vi"("Name"=w381) -> ("String"=w380:string)  [unwired: 9 in, 1 out]
                n227 = Unbundle(w379) -> (w376:string[])
                n228 = Match First String(2:w376, 3:w380) -> (0:w375:i32)  [unwired: 1 out]
                n229 = property on="Test Ring" class="Ring (strict)"("Value"=w375, "Strings []"=w376) -> ()  [unwired: 2 in, 2 out]
                n230 = property on="Test Ring" class="Ring (strict)"("Visible"=TRUE) -> ()  [unwired: 2 in, 2 out]
                n231 = property on="Test Slider" class="Slide (strict)"("Visible"=FALSE) -> ()  [unwired: 2 in, 2 out]
              }
              frame "Exposure  **" {
                n232 = Index Array(array=w387, index=2) -> (element=w388:cluster{string[]})
                n233 = call <vilib>:"NT Read String.vi"("Name"=w390) -> ("String"=w389:string)  [unwired: 9 in, 1 out]
                n234 = Unbundle(w388) -> (w384:string[])
                n235 = Match First String(2:w384, 3:w389) -> (0:w385:i32)  [unwired: 1 out]
                n236 = property on="Test Ring" class="Ring (strict)"("Value"=w385, "Strings []"=w384) -> ()  [unwired: 2 in, 2 out]
                n237 = property on="Test Ring" class="Ring (strict)"("Visible"=TRUE) -> ()  [unwired: 2 in, 2 out]
                n238 = property on="Test Slider" class="Slide (strict)"("Visible"=FALSE) -> ()  [unwired: 2 in, 2 out]
              }
              frame "Exposure Priority  **" {
                n239 = Index Array(array=w396, index=3) -> (element=w397:cluster{string[]})
                n240 = call <vilib>:"NT Read String.vi"("Name"=w399) -> ("String"=w398:string)  [unwired: 9 in, 1 out]
                n241 = Unbundle(w397) -> (w393:string[])
                n242 = Match First String(2:w393, 3:w398) -> (0:w394:i32)  [unwired: 1 out]
                n243 = property on="Test Ring" class="Ring (strict)"("Value"=w394, "Strings []"=w393) -> ()  [unwired: 2 in, 2 out]
                n244 = property on="Test Ring" class="Ring (strict)"("Visible"=TRUE) -> ()  [unwired: 2 in, 2 out]
                n245 = property on="Test Slider" class="Slide (strict)"("Visible"=FALSE) -> ()  [unwired: 2 in, 2 out]
              }
              frame "Color Enable  **" {
                n246 = Index Array(array=w405, index=4) -> (element=w406:cluster{string[]})
                n247 = call <vilib>:"NT Read String.vi"("Name"=w408) -> ("String"=w407:string)  [unwired: 9 in, 1 out]
                n248 = Unbundle(w406) -> (w402:string[])
                n249 = Match First String(2:w402, 3:w407) -> (0:w403:i32)  [unwired: 1 out]
                n250 = property on="Test Ring" class="Ring (strict)"("Value"=w403, "Strings []"=w402) -> ()  [unwired: 2 in, 2 out]
                n251 = property on="Test Ring" class="Ring (strict)"("Visible"=TRUE) -> ()  [unwired: 2 in, 2 out]
                n252 = property on="Test Slider" class="Slide (strict)"("Visible"=FALSE) -> ()  [unwired: 2 in, 2 out]
              }
              frame Default {
                n253 = property on="Test Ring" class="Ring (strict)"("Visible"=FALSE) -> ()  [unwired: 2 in, 2 out]
                n254 = property on="Test Slider" class="Slide (strict)"("Visible"=FALSE) -> ()  [unwired: 2 in, 2 out]
              }
              frame "Brightness  **", "Color Level  **", "Compression  **", "FPS  **", "Sharpness  **" {
                n255 = call <vilib>:"NT Read Number.vi"("Name"=w414) -> ("Numeric"=w413:dbl)  [unwired: 9 in, 1 out]
                n256 = local write "Test Slider"(w413) -> ()
                n257 = property on="Test Slider" class="Slide (strict)"("Visible"=TRUE, "Scale.Maximum"=100.0 ("Scale.Range:Maximum")) -> ()  [unwired: 2 in, 2 out]
                n258 = property on="Test Ring" class="Ring (strict)"("Visible"=FALSE) -> ()  [unwired: 2 in, 2 out]
              }
            }
          }
        }
        n259 = property on="Progress" class="Clust (strict)"("Visible"=FALSE) -> ()  [unwired: 2 in, 2 out]
      }
      event "Test Name": Mouse Enter {
        # "Populate the ring with the list of tests"
        n260 = event-data() -> ()  [unwired: 1 in, 1 out]
        n261 = call <vilib>:"NT Read String Array.vi"("Name"="/TestMode/TestList") -> ("String Array"=w422:string[])  [unwired: 9 in, 1 out]
        n262 = Build Array (concatenate)("Select the test to run...", w422) -> (w421:string[])
        n263 = property on="Test Name" class="Ring (strict)"("Strings []"=w421) -> ()  [unwired: 2 in, 2 out]
      }
      event "Test Name": Value Change {
        w424 = FALSE ("Visible")
        # "Tell the robot the test name to run"
        n264 = event-data() -> ("NewVal"=w428:u16)  [unwired: 1 in]
        n265 = property on="Test Name" class="Ring (strict)"() -> ("Strings []"=w429:string[])  [unwired: 2 in, 2 out]
        n266 = local write "Progress"(T6 {"Test Progress"=0, "Test Progress Text"=""} ("Progress")) -> ()
        n267 = Index Array(array=w429, index=w428) -> (element=w427:string)
        n268 = call <vilib>:"NT Write String.vi"("String"=w427, "Name"="/TestMode/TestName") -> ()  [unwired: 9 in, 1 out]
        n269 = property on="Progress" class="Clust (strict)"("Visible"=TRUE) -> ()  [unwired: 2 in, 2 out]
        n270 = property on="Motor" class="Clust (strict)"("Visible"=w424) -> ()  [unwired: 2 in, 2 out]
        n271 = property on="Test Slider" class="Slide (strict)"("Visible"=w424) -> ()  [unwired: 2 in, 2 out]
        n272 = property on="On/Off" class="Bool (strict)"("Visible"=w424) -> ()  [unwired: 2 in, 2 out]
        n273 = property on="Rev/Fwd" class="Clust (strict)"("Visible"=w424) -> ()  [unwired: 2 in, 2 out]
        n274 = property on="Test Ring" class="Ring (strict)"("Visible"=w424) -> ()  [unwired: 2 in, 2 out]
      }
      event "Select Auto": Mouse Enter {
        # "Populate the combo box with the list of autonomous options"
        n275 = event-data() -> ()  [unwired: 1 in, 1 out]
        n276 = call <vilib>:"NT Read String Array.vi"("Name"="Auto List") -> ("String Array"=w431:string[])  [unwired: 9 in, 1 out]
        n277 = property on="Select Auto" class="CmbBox"("Strings[]"=w431) -> ()  [unwired: 2 in, 2 out]
      }
      event "Select Auto": Value Change {
        # "User modified the Auto Selection. Write to NT variable so robot knows."
        n278 = event-data() -> ("NewVal"=w434:string)  [unwired: 1 in]
        n279 = call <vilib>:"NT Write String.vi"("String"=w434, "Name"="Auto Selector") -> ()  [unwired: 9 in, 1 out]
      }
      event "Command Selection": Value Change {
        # "Get the params and show in table"
        n280 = event-data() -> ("NewVal"=w440:i32)  [unwired: 1 in]
        n281 = property on="Command Selection" class="MCListbox (strict)"() -> ("ItemNames"=w438:string[][])  [unwired: 2 in, 2 out]
        n282 = call <vilib>:"WPI_DashboardUpdate Command Params.vi"("NewVal"=w440, "Commands"=w438, "Param Tbl"=w439) -> ()  [unwired: 8 in, 1 out]
      }
      event "Execute Command": Value Change {
        # "Started one, Unique ID holds\nresponse"
        n283 = event-data() -> ()  [unwired: 1 in, 1 out]
        n284 = property on="Command Selection" class="MCListbox (strict)"() -> ("ItemNames"=w451:string[][])  [unwired: 2 in, 2 out]
        n285 = Index Array(array=w451, index (row)="Command Selection", index (col)=0) -> (element=w449:string)
        n286 = call <vilib>:"Invoke Commands.vi"("Command Params"="Command Params", "Function Name"=w449) -> ("Params"=w445:u8, "Started"=w444:bool)  [unwired: 7 in, 1 out]
        n287 = Array Subset(array="Command Params", length (row)=w445) -> (w446:string[][])  [unwired: 3 in]
        n288 = Select(t="Executing" ("Cmd Status"), s=w444, f="" ("Cmd Status")) -> (s? t:f=→"Cmd Status":string)
      }
      event "Command Selection": Double Click {
        n289 = event-data() -> ("Row"=w459:i32)  [unwired: 1 in]
        n290 = property on="Command Selection" class="MCListbox (strict)"() -> ("ItemNames"=w462:string[][])  [unwired: 2 in, 2 out]
        n291 = local read "Command Params"() -> (w458:string[][])
        n292 = Index Array(array=w462, index (row)=w459, index (col)=0) -> (element=w460:string)
        n293 = call <vilib>:"Invoke Commands.vi"("Command Params"=w458, "Function Name"=w460) -> ("Params"=w457:u8, "Started"=w452:bool)  [unwired: 7 in, 1 out]
        n294 = Array Subset(array=w458, length (row)=w457) -> (w456:string[][])  [unwired: 3 in]
        n295 = Select(t="Executing" ("Cmd Status"), s=w452, f="" ("Cmd Status")) -> (s? t:f=w453:string)
        n296 = local write "Cmd Status"(w453) -> ()
      }
      event "CheckList": Double Click {
        # "Shift clears all"
        # "Update symbols on the listbox"
        n297 = event-data() -> ("PlatMods.Shift"=w464:bool, "Row"=w466:i32)  [unwired: 1 in]
        n298 = case shown="True" w464 {
          tunnel: w466 -> [w470 _]
          tunnel: 1 -> [w469 _]
          frame False {
            n299 = property on="CheckList" class="LstBox (strict)"() -> ("Item Symbols"=w468:i32[])  [unwired: 2 in, 2 out]
            n300 = Replace Array Subset(array=w468, new element=w469, index=w470) -> (w467:i32[])
            n301 = property on="CheckList" class="LstBox (strict)"("Item Symbols"=w467) -> ()  [unwired: 2 in, 2 out]
          }
          frame True {
            w471 = 0 ("Top Row")
            n302 = property on="CheckList" class="LstBox (strict)"() -> ("Number of Rows"=w473:u32)  [unwired: 2 in, 2 out]
            n303 = Initialize Array(0, w473) -> (w472:i32[])
            n304 = property on="CheckList" class="LstBox (strict)"("Top Row"=w471, "Value"=w471, "Item Symbols"=w472) -> ()  [unwired: 2 in, 2 out]
          }
        }
      }
      event "CheckList": Key Down {
        # "Update symbols on the listbox\nLeft and right keys check and uncheck"
        n305 = event-data() -> ("VKey"=w477:T20)  [unwired: 1 in]
        n306 = case shown="\"Left\", \"Right\"" w477 {
          selector: w477 -> [w482 _]
          tunnel: eventvkey."Left" ("VKey") -> [w480 _]
          frame "Left", "Right" {
            n307 = Equal?(x=w480, y=w482) -> (x = y?=w481:bool)
            n308 = Select(t=0, s=w481, f=1) -> (s? t:f=w483:i32)
            n309 = property on="CheckList" class="LstBox (strict)"() -> ("Item Symbols"=w486:i32[])  [unwired: 2 in, 2 out]
            n310 = Replace Array Subset(array=w486, new element=w483, index="CheckList") -> (w485:i32[])
            n311 = property on="CheckList" class="LstBox (strict)"("Item Symbols"=w485) -> ()  [unwired: 2 in, 2 out]
          }
          frame Default {
          }
        }
      }
      event "Motor.Enable": Value Change {
        # "When the test mode otor enable helper is set, update that\ntree row item's value"
        n312 = event-data() -> ("NewVal"=w492:bool)  [unwired: 1 in]
        n313 = Unbundle("Motor") -> ("Value"=w491:dbl)  [unwired: 1 out]
        n314 = Select(t=w491, s=w492, f=0.0) -> (s? t:f=w489:dbl)
        n315 = call <vilib>:"NT Write Number.vi"("Numeric"=w489, "Name"=w488) -> ()  [unwired: 9 in, 1 out]
      }
      event "Test Slider": Value Change {
        # "When the test mode slider helper is set, update that\ntree row item's value"
        n316 = event-data() -> ("NewVal"=w497:dbl)  [unwired: 1 in]
        n317 = Not Equal?(x=w500, y="ElevatorMtr") -> (x != y?=w498:bool)
        n318 = Absolute Value(x=w497) -> (abs(x)=w496:dbl)
        n319 = Negate(x=w496) -> (-x=w495:dbl)
        n320 = Select(t=w497, s=w498, f=w495) -> (s? t:f=w494:dbl)
        n321 = call <vilib>:"NT Write Number.vi"("Numeric"=w494, "Name"=w500) -> ()  [unwired: 9 in, 1 out]
      }
      event "On/Off": Value Change {
        # "When the test mode on/off helper value is set, update that\ntree row item's value"
        n322 = event-data() -> ("NewVal"=w505:bool)  [unwired: 1 in]
        n323 = Boolean To (0,1)(Boolean=w505) -> (0, 1=w504:i16)
        n324 = call <vilib>:"NT Write Number.vi"("Numeric"=w504, "Name"=w503) -> ()  [unwired: 9 in, 1 out]
      }
      event "Rev/Fwd": Value Change {
        # "When the test mode helper value for relays is set, update that\ntree row item's value"
        n325 = event-data() -> ("NewVal.Forward"=w513:bool, "NewVal.Reverse"=w512:bool)  [unwired: 1 in]
        n326 = Boolean To (0,1)(Boolean=w513) -> (0, 1=w509:i16)
        n327 = Boolean To (0,1)(Boolean=w512) -> (0, 1=w511:i16)
        n328 = Negate(x=w511) -> (-x=w510:i16)
        n329 = Add(x=w509, y=w510) -> (x+y=w508:i16)
        n330 = call <vilib>:"NT Write Number.vi"("Numeric"=w508, "Name"=w507) -> ()  [unwired: 9 in, 1 out]
      }
      event "Test Ring": Value Change {
        # "When a test mode helper value is selected from the ring,\nset the tree item's variable to the string value"
        n331 = event-data() -> ("NewVal"=w517:u16)  [unwired: 1 in]
        n332 = property on="Test Ring" class="Ring (strict)"() -> ("Strings []"=w518:string[])  [unwired: 2 in, 2 out]
        n333 = Index Array(array=w518, index=w517) -> (element=w516:string)
        n334 = call <vilib>:"NT Write String.vi"("String"=w516, "Name"=w515) -> ()  [unwired: 9 in, 1 out]
      }
      event "Rec Mode": Value Change {
        # "Update globals for recording mode and path to read log from.\nClear when logging and let NetworkTables set path for vision to\nuse."
        n335 = event-data() -> ("NewVal"=w529:enum32{"Stop", "Record", "Playback"})  [unwired: 1 in]
        n336 = global write "WPI_DashboardLogging Global.vi" "Logging Filename"(path "") -> ()
        n337 = global write "WPI_DashboardLogging Global.vi" "Recording"(w529) -> ()
        n338 = case shown="\"Playback\"" w529 {
          tunnel: w528 -> [_ w531 w540]
          tunnel: [_ _ w539] -> w526
          tunnel: [_ _ w538] -> _
          tunnel: w524 -> [_ _ w536]
          tunnel: cluster{i32, i32} {-250, 170} -> [_ _ w535]
          tunnel: [_ _ T21 {"Image Size"=TRUE, "Image Type"=TRUE, "Pixel Value"=TRUE, "ROI Information"=TRUE, "Zoom Factor"=FALSE} ("Image Information Shown:All Elements")] -> w522
          tunnel: [_ _ TRUE ("Zoom Factor")] -> w521
          tunnel: w520 -> [_ _ w532]
          frame Default {
          }
          frame "Stop", "Record" {
            # "Place Window too"
            n339 = invoke class="VI" method="FP.Close"(reference=w531) -> (reference out=w530:refnum<vi>)  [unwired: 2 in, 2 out]
            n340 = invoke class="VI" method="Abort VI"(reference=w530) -> ()  [unwired: 2 in, 3 out]
          }
          frame "Playback" {
            n341 = call "Open Playback Panel.vi"("Offset"=w535, "DB VI Ref"=w536, "Playback in"=w540) -> ("Playback out"=w537:refnum<vi>)  [unwired: 8 in]
            n342 = register-events(w537, w532) -> (reference out=w539:refnum<event-registration>, error out=w538:errorcluster)  [unwired: 2 in]
          }
        }
        n343 = property on="Camera Image" class="ImageControl"("Image Information Shown"=w522, "Image Information Visible"=w521) -> ()  [unwired: 2 in, 2 out]
        n344 = call <vilib>:"WPI_DashboardNT Log FieldName Cache.vi"("Operation"=enum16{"Lookup/Add", "Index", "Clear"}."Clear") -> ()  [unwired: 8 in, 3 out]
      }
      event Panel Close {
        w542 = enum32{"Stop", "Record", "Playback"}."Stop" ("Rec Mode")
        # "Playback window has been closed, abort"
        n345 = event-data() -> ()  [unwired: 1 in, 4 out]
        n346 = local write "Rec Mode"(w542) -> ()
        n347 = global write "WPI_DashboardLogging Global.vi" "Recording"(w542) -> ()
      }
      event Panel Close {
        # "Abort playback window and ourself"
        n348 = event-data() -> ()  [unwired: 1 in, 4 out]
        n349 = invoke class="VI" method="FP.Close"(reference=w546) -> (reference out=w545:refnum<vi>)  [unwired: 2 in, 2 out]
        n350 = invoke class="VI" method="Abort VI"(reference=w545) -> (error out=w544:errorcluster)  [unwired: 2 in, 2 out]
        n351 = invoke class="VI" method="Abort VI"(error in=w544) -> ()  [unwired: 2 in, 3 out]
      }
      event User Event {
        n352 = event-data() -> ("IDs"=w553:cluster{"RPC field ID":u16, "Unique ID":u16}, "String"=w552:string)  [unwired: 1 in]
        n353 = Bundle("IDs"=w553, "String"=w552) -> (w551:T8)  [unwired: 1 in]
        n354 = call <vilib>:"Retrieve RPC Response.vi"("RPC Response"=w551) -> ("Output"=w549:string[][])  [unwired: 10 in]
        n355 = Build Array (concatenate)(w547, w549) -> (w548:string[][])
        n356 = local write "Command Params"(w548) -> ()
        n357 = local write "Cmd Status"("" ("Cmd Status")) -> ()
      }
      event "Tree": Double Click {
        n358 = event-data() -> ("PlatMods"=w557:T24, "Tag"=w556:string)  [unwired: 1 in]
        n359 = Unbundle(w557) -> ("Shift"=w555:bool)  [unwired: 4 out]
        n360 = Not(x=w555) -> (.not. x?=w554:bool)
        n361 = call <vilib>:"NT Update Persistence.vi"("Persistence"=w554, "Name"=w556) -> ()  [unwired: 9 in, 1 out]
      }
    }
  }
  n362 = while {
    tunnel: w64 -> [w560]
    i -> [w563]
    stop <- FALSE stop-if-true
    n363 = Wait (ms)(milliseconds to wait=u32 100) -> ()  [unwired: 1 out]
    n364 = case shown="\"Playback\"" "Rec Mode" {
      tunnel: w563 -> [_ _ w578]
      tunnel: [u32 2829099 ("Base Color") u32 11141120 ("Target Color") w567] -> w559
      frame "Stop", Default {
        # "Reset the color, extra updates don't cost much"
      }
      frame "Record" {
      }
      frame "Playback" {
        # "Playback"
        n365 = Quotient & Remainder(x=w578, y=u32 50 ("milliseconds to wait")) -> (x-y*floor(x/y)=w574:u32)  [unwired: 1 out]
        n366 = Divide(x=w574, y=u32 50 ("milliseconds to wait")) -> (x/y=w571:dbl)
        n367 = Multiply(x=6.283185307179586, y=w571) -> (x*y=w576:dbl)
        n368 = Sine(x=w576) -> (sin(x)=w575:dbl)
        n369 = Absolute Value(x=w575) -> (abs(x)=w568:dbl)
        n370 = call "Interpolate RGB Color.vi"("Proportion"=w568, "Target Color"=u32 30976, "Base Color"=u32 2829099) -> ("Result Color"=w567:u32)  [unwired: 8 in]
      }
    }
    n371 = property class="Pane"(reference=w560, "PaneColor"=w559) -> ()  [unwired: 1 in, 2 out]
  }
  n372 = local write "Dashboard Tab"(T9."Drive" ("Dashboard Tab")) -> ()
  n373 = property on="On/Off" class="Bool (strict)"("Visible"=w33) -> ()  [unwired: 2 in, 2 out]
  n374 = property on="Motor" class="Clust (strict)"("Visible"=w33) -> ()  [unwired: 2 in, 2 out]
  n375 = property on="Progress" class="Clust (strict)"("Visible"=w33) -> ()  [unwired: 2 in, 2 out]
  n376 = property on="Test Ring" class="Ring (strict)"("Visible"=w33) -> ()  [unwired: 2 in, 2 out]
  n377 = property on="Rev/Fwd" class="Clust (strict)"("Visible"=w33) -> ()  [unwired: 2 in, 2 out]
  n378 = local write "Command Selection"(u16 0 ("milliseconds to wait")) -> ()
  n379 = while {
    tunnel: u16 1741 ("timeout ms (25000)") -> [w580]
    stop <- FALSE stop-if-true
    n380 = TCP Create Listener(10:w580) -> (0:w579:errorcluster, 3:w581:refnum<k5>)  [unwired: 4 in, 1 out]
    n381 = case shown="No Error" w579 {
      selector: w579 -> [w583 _]
      tunnel: w581 -> [w584 _]
      frame No Error {
        n382 = while {
          tunnel: w584 -> [w587]
          tunnel: w583 -> [w586]
          stop <- FALSE stop-if-true
          n383 = TCP Wait On Listener(8:w586, 11:w587) -> (0:w588:errorcluster, 4:w589:refnum<k5>)  [unwired: 2 in, 3 out]
          n384 = local write "TCP"(w589) -> ()
          n385 = case shown="No Error" w588 {
            frame No Error {
            }
            frame Error {
              n386 = Wait (ms)(milliseconds to wait=u32 1000) -> ()  [unwired: 1 out]
            }
          }
        }
      }
      frame Error {
        n387 = Wait (ms)(milliseconds to wait=u32 1000) -> ()  [unwired: 1 out]
      }
    }
  }
  n388 = local write "Command Params"(string[][] [] ("Command Params")) -> ()
  n389 = global write "WPI_DashboardLogging Global.vi" "Recording"(w58) -> ()
  n390 = local write "Rec Mode"(w58) -> ()
  n391 = call <vilib>:"NT Write String.vi"("String"="Select Auto", "Name"="Auto Selector") -> ()  [unwired: 9 in, 1 out]
